vi "Simulate_kafkaStream_Write.vi"(0 "Kafka Producer Handle":string, 1 "File Name":string="untitled", 2 "Kafka Partition":u32, 5 "Group Name":string, 7 "Channel Names":string[](array[string]), 9 "Waveforms":waveform(dbl)[](array[waveform]), 11 "error in (no error)":errorcluster) -> (3 "File Name Out":string="untitled", 4 "Kafka Producer Handle Out":string, 6 "Group Name Out":string, 8 "Channel Names Out":string[](array[string]), 15 "error out":errorcluster)   [LabVIEW 2019]
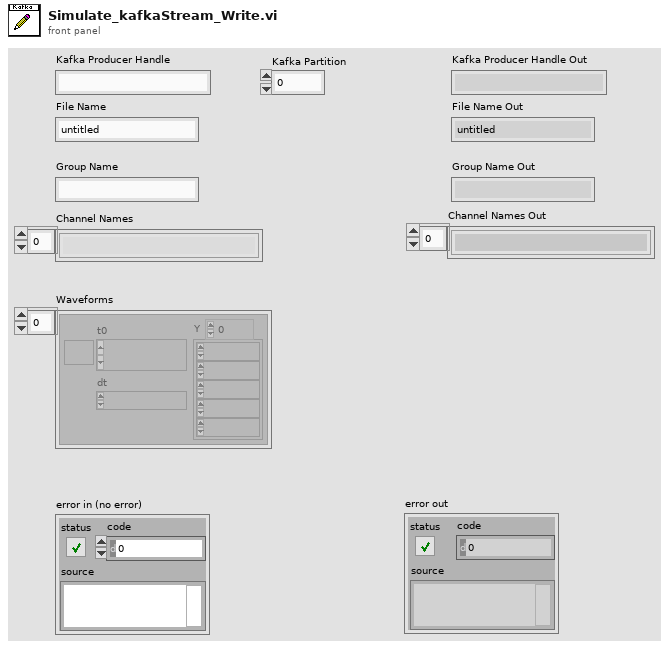
[diagram p1: front panel]
types:
  T1 = typedef "KafkaConsumerEvent.ctl" = cluster{"Payload":string, "Key":string, "MsgLen":u64, "Offset":i64, "Time Stamp":i64, "TS Name":string}
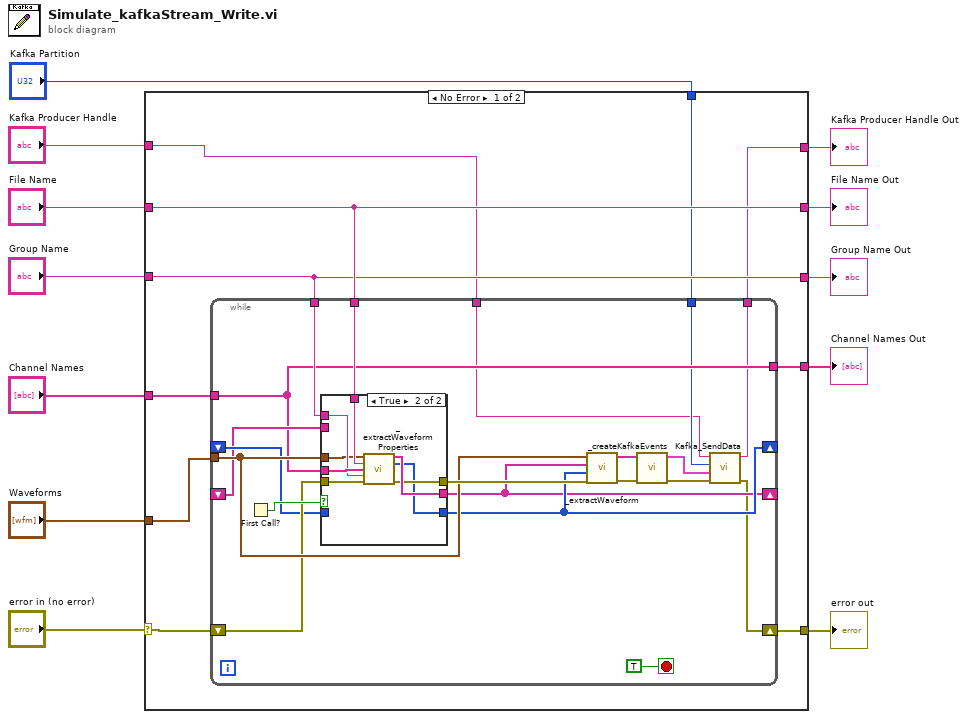
[diagram p0: block diagram]
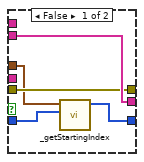
[diagram p2: hidden frame]
diagram:
  n1 = case shown="No Error" "error in (no error)" {
    selector: "error in (no error)" -> [w22 w60]
    tunnel: "Group Name" -> [w17 w58]
    tunnel: "Channel Names" -> [w19 w59]
    tunnel: "Waveforms" -> [w20 _]
    tunnel: [w21 w60] -> w8
    tunnel: "File Name" -> [w18 w57]
    tunnel: [w16 w59] -> w6
    tunnel: [w17 w58] -> w5
    tunnel: [w18 w57] -> w4
    tunnel: "Kafka Partition" -> [w15 _]
    tunnel: "Kafka Producer Handle" -> [w14 w56]
    tunnel: [w13 w56] -> w1
    frame No Error {
      n2 = while {
        shift-right: [w26] -> w21
        shift-left: w22 -> [w38]
        tunnel: w20 -> [w39]
        tunnel: w19 -> [w31]
        tunnel: w17 -> [w37]
        shift-right: [w36] -> _
        shift-left: _ -> [w35]
        shift-right: [w34] -> _
        shift-left: _ -> [w33]
        tunnel: w18 -> [w32]
        tunnel: [w31] -> w16
        tunnel: w15 -> [w28]
        tunnel: w14 -> [w27]
        tunnel: [w23] -> w13
        stop <- TRUE stop-if-true
        n3 = First Call?() -> (First Call?: T/F=w41:bool)
        n4 = case shown="True" w41 {
          tunnel: w39 -> [w45 w49]
          tunnel: w38 -> [w46 w55]
          tunnel: w31 -> [_ w54]
          tunnel: w37 -> [_ w52]
          tunnel: w32 -> [_ w53]
          tunnel: [w47 w51] -> w34
          tunnel: w33 -> [w47 _]
          tunnel: [w46 w50] -> w42
          tunnel: [w44 w48] -> w36
          tunnel: w35 -> [w43 _]
          frame False {
            n5 = call "_getStartingIndex.vi"("Starting Index In"=w43, "Waveforms"=w45) -> ("Starting Index"=w44:u32[])  [unwired: 9 in]
          }
          frame True {
            n6 = call "_extractWaveformProperties.vi"("Waveforms"=w49, "File Name"=w53, "Channel Names"=w54, "Group Name"=w52, "error in (no error)"=w55) -> ("Event Object"=w51:string[], "Starting Index Increment"=w48:u32[], "error out"=w50:errorcluster)  [unwired: 8 in]
          }
        }
        n7 = call "_extractWaveform.vi"("Waveforms"=w39, "Event Object In"=w34, "Starting Index"=w36, "error in (no error)"=w42) -> ("Event Object Out"=w24:string[], "error out"=w25:errorcluster)  [unwired: 5 in]
        n8 = call "_createKafkaEvents.vi"("Payload"=w24, "error in (no error)"=w25) -> ("Kafka Events"=w30:T1[], "error out"=w29:errorcluster)  [unwired: 7 in]
        n9 = call "Kafka_SendData.vi"("error in (no error)"=w29, "Events"=w30, "Partition"=w28, "Producer Handle"=w27) -> ("error out"=w26:errorcluster, "Producer Handle"=w23:string)  [unwired: 6 in]
      }
    }
    frame Error {
    }
  }
  "error out" <- w8
  "Channel Names Out" <- w6
  "Group Name Out" <- w5
  "File Name Out" <- w4
  "Kafka Producer Handle Out" <- w1
